vi "ShotDateTimeToNode(viaString).vi"(7 "DateTime Path":string, 8 "error in":errorcluster, 11 "Tree DVR in":refnum<data-value>) -> (0 "error out":errorcluster)   [LabVIEW 2014]
uses:
  <vilib>/MDSplus/Classes/Tree_Class/Tree.lvclass
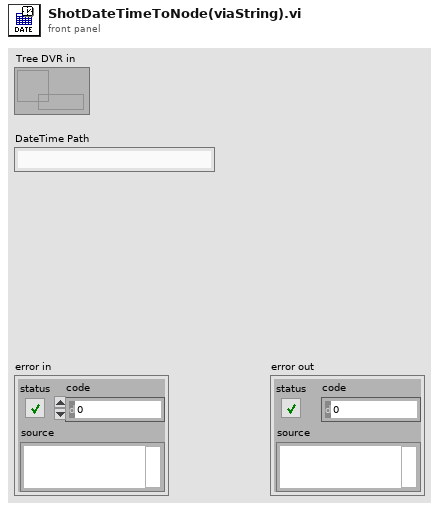
[diagram p1: front panel]
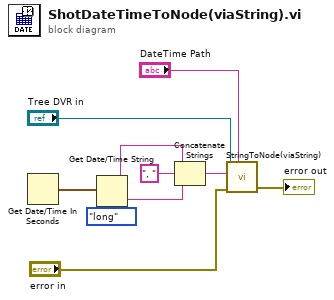
[diagram p0: block diagram]
diagram:
  n1 = Get Date/Time In Seconds() -> (seconds since 1Jan1904=w1:timestamp)
  n2 = Get Date/Time String(date format (0)=enum16{"short", "long", "abbreviated"}."long", seconds (now)=w1) -> (date string=w7:string, time string=w6:string)  [unwired: 1 in]
  n3 = Concatenate Strings(w7, ", " ("string"), w6) -> (w8:string)
  n4 = call "StringToNode(viaString).vi"("Tree DVR in"="Tree DVR in", "String value in"=w8, "error in (no error)"="error in", "NodePath"="DateTime Path") -> ("error out"=→"error out":errorcluster)  [unwired: 1 in, 2 out]
